vi "Move.vi"(8 "error in (no error)":errorcluster, 11 "StageSPIM in":refnum<class "StageSPIM.lvclass">) -> (0 "error out":errorcluster, 3 "StageSPIM out":refnum<class "StageSPIM.lvclass">)   [LabVIEW 2012, in "StageSPIM.lvclass"]
uses:
  StageSPIM.lvclass
  StageSPIM.lvclass/StageSPIM.ctl
panel:
  out "Target position":dbl[][](array[numeric])
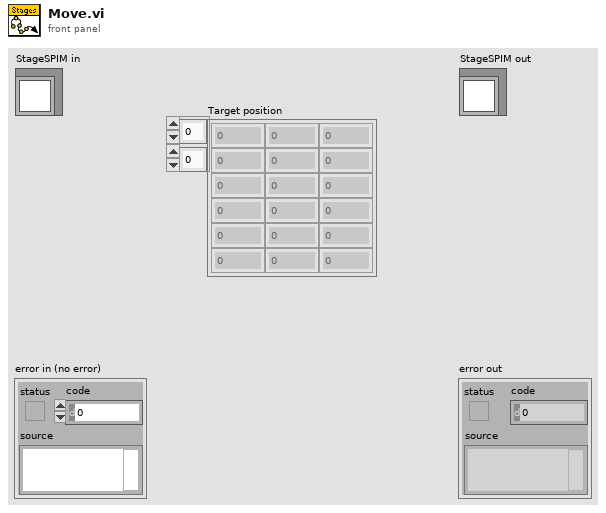
[diagram p1: front panel]
types:
  T1 = typedef "Semaphore RefNum" = refnum<k1>
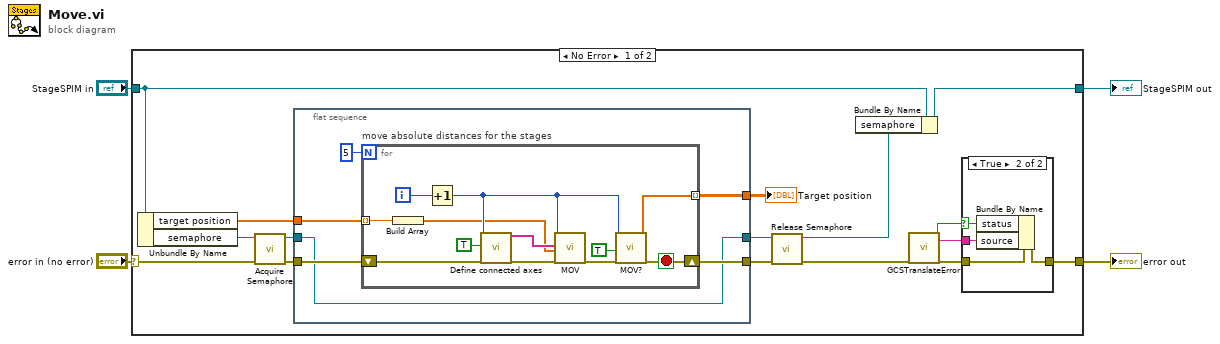
[diagram p0: block diagram]
diagram:
  n1 = case shown="No Error" "error in (no error)" {
    selector: "error in (no error)" -> [w20 w45]
    tunnel: [w17 w45] -> w3
    tunnel: [w8 w44] -> w1
    tunnel: "StageSPIM in" -> [w9 w44]
    frame No Error {
      n2 = Unbundle By Name(w9) -> ("target position"=w19:dbl[], "semaphore"=w11:T1)
      n3 = call <vilib>:"Acquire Semaphore.vi"("error in (no error)"=w20, "semaphore"=w11) -> ("error out"=w12:errorcluster, "semaphore out"=w5:T1)  [unwired: 3 in, 1 out]
      n4 = flat-sequence {
        tunnel: w19 -> [w25]
        tunnel: [w24] -> w14
        tunnel: [w23] -> w13
        tunnel: w12 -> [w22]
        tunnel: [w21] -> w6
        tunnel: w5 -> [w21]
        frame #0 {
          n5 = for "move absolute distances for the stages" {
            N: 5 -> [_]
            shift-right: [w28] -> w23
            shift-left: w22 -> [w37]
            tunnel: w25 -> [w38] mode=indexing
            tunnel: [w27] -> w24 mode=indexing
            i -> [w36]
            stop <- w28 stop-if-true
            n6 = Build Array(w38) -> (w30:dbl[])
            n7 = Increment(x=w36) -> (x+1=w35:i32)
            n8 = call "Define connected axes.vi"("System no."=w35, "Read from\ncontroller?"=TRUE ("Read from\ncontroller?"), "error in"=w37) -> ("Conn. Axes out"=w31:string[], "error out"=w34:errorcluster)  [unwired: 15 in]
            n9 = call "MOV.vi"("System no."=w35, "Axes to move"=w31, "Position values"=w30, "error in"=w34) -> ("error out"=w33:errorcluster)  [unwired: 15 in]
            n10 = call "MOV?.vi"("System no."=w35, "All axes?"=TRUE, "error in"=w33) -> ("Target position"=w27:dbl[], "error out"=w28:errorcluster)  [unwired: 15 in]
          }
        }
      }
      n11 = call <vilib>:"Release Semaphore.vi"("error in (no error)"=w13, "semaphore"=w6) -> ("error out"=w10:errorcluster, "semaphore out"=w7:T1)  [unwired: 4 in]
      n12 = Bundle By Name(cluster=w9, "semaphore"=w7) -> (w8:refnum<class "StageSPIM.lvclass">)
      n13 = call "GCSTranslateError.vi"("error in"=w10) -> ("GCS Error?"=w16:bool, "Error Description"=w15:string, "error out"=w18:errorcluster)  [unwired: 16 in]
      n14 = case shown="True" w16 {
        selector: w16 -> [_ w41]
        tunnel: w18 -> [w39 w43]
        tunnel: [w39 w42] -> w17
        tunnel: w15 -> [_ w40]
        frame False {
        }
        frame True {
          n15 = Bundle By Name(cluster=w43, "status"=w41, "source"=w40) -> (w42:errorcluster)
        }
      }
      "Target position" <- w14
    }
    frame Error {
    }
  }
  "error out" <- w3
  "StageSPIM out" <- w1
